vi "单体信息全局.vi"() -> ()   [LabVIEW 2013]
panel:
  out "数据":dbl[](array[numeric])
  out "温度数据":u8[][](array[numeric])
  out "SOC位置":i32[](array[numeric])
  out "均衡PF":i32=48
  out "均衡故障":dbl[](array[numeric])
  out "充电均衡":dbl[](array[numeric])
  out "放电均衡":dbl[](array[numeric])
  out "PF2":i32
  out "PF":i32
  out "数据 2":dbl[](array[numeric])
  out "位置 2":i32[](array[numeric])
  out "单体数据":dbl[][](array[numeric])
  out "位置":i32[](array[numeric])
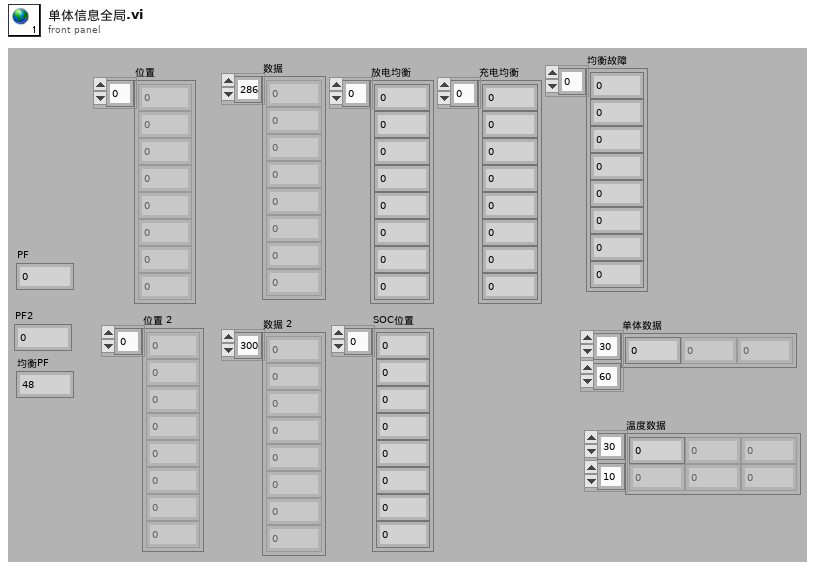
[diagram p1: front panel]
diagram:
